vi "Sub_CalculateArrayAverage.vi"(1 "Array to be averaged":dbl[](array[numeric])) -> (0 "Average":dbl)   [LabVIEW 2021]
panel:
  # "Inputs"
  # "Outputs"
  # "Required:"
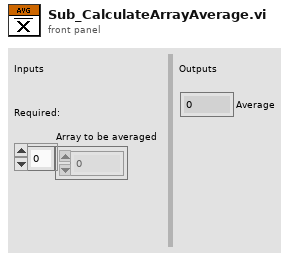
[diagram p1: front panel]
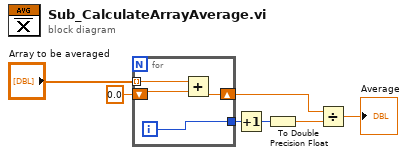
[diagram p0: block diagram]
diagram:
  n1 = for {
    tunnel: "Array to be averaged" -> [w9] mode=indexing
    shift-right: [w10] -> w5
    shift-left: 0.0 ("Numeric") -> [w8]
    tunnel: [w11] -> w4
    i -> [w11]
    n2 = Add(x=w9, y=w8) -> (x+y=w10:dbl)
  }
  n3 = Increment(x=w4) -> (x+1=w3:i32)
  n4 = To Double Precision Float(number=w3) -> (double precision float=w2:dbl)
  n5 = Divide(x=w5, y=w2) -> (x/y=→"Average":dbl)
